vi "Temp from Voltage Calculator.vi"(8 "error in (no error)":errorcluster, 9 "Calibrations":dbl[](array[numeric]), 10 "Thermistor":T1, 11 "Data_Array":dbl[](array[numeric])) -> (1 "Temp Filtered":dbl[](array[numeric]), 2 "Temp":dbl[](array[numeric]), 3 "Time Read":timestamp[](array[timestamp]), 4 "error out":errorcluster[](array[cluster]))   [LabVIEW 2021]
uses:
  <vilib>/express/express arith-compare/Formula/XNode/ExpressFormulaBlockNode.xnode
  <vilib>/ptbypt/NI_PtbyPt.lvlib
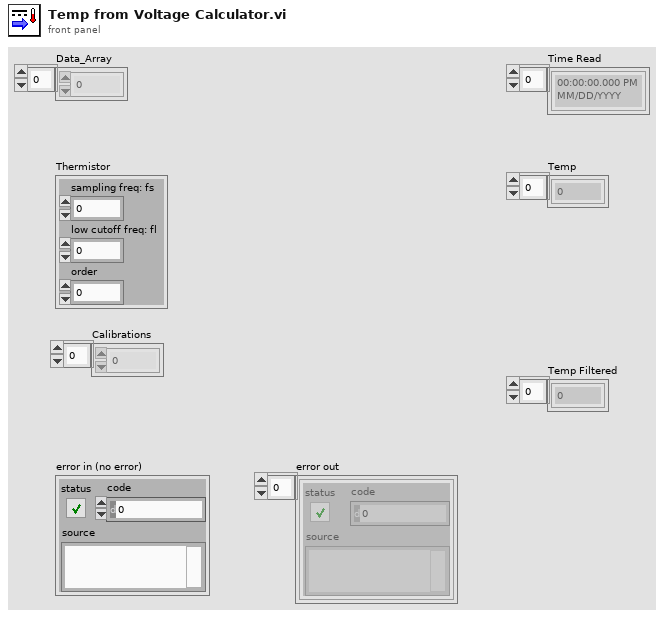
[diagram p1: front panel]
types:
  T1 = cluster{"sampling freq: fs":dbl, "low cutoff freq: fl":dbl, "order":i32}
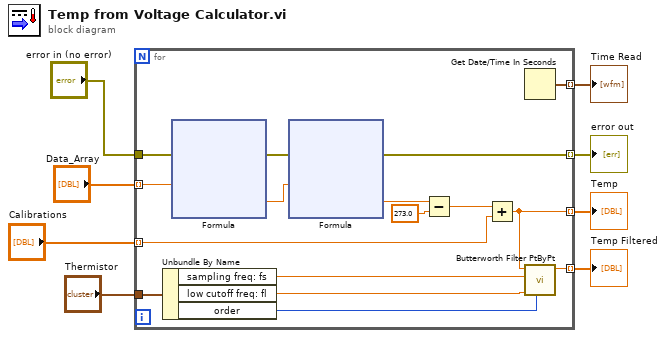
[diagram p0: block diagram]
diagram:
  n1 = for {
    tunnel: "Data_Array" -> [w19] mode=indexing
    tunnel: "Thermistor" -> [w18]
    tunnel: [w14] -> w4 mode=indexing
    tunnel: [w17] -> w8 mode=indexing
    tunnel: [w15] -> w7 mode=indexing
    tunnel: "error in (no error)" -> [w12]
    tunnel: [w10] -> w6 mode=indexing
    tunnel: "Calibrations" -> [w9] mode=indexing
    n2 = Unbundle By Name(w18) -> ("sampling freq: fs"=w23:dbl, "low cutoff freq: fl"=w22:dbl, "order"=w21:i32)
    n3 = xnode "Formula"("v"=w19, "error in (no error)"=w12) -> ("Result"=w13:dbl, "error out"=w11:errorcluster)
    n4 = xnode "Formula"("R"=w13, "error in (no error)"=w11) -> ("Result"=w20:dbl, "error out"=w10:errorcluster)
    n5 = Subtract(x=w20, y=273.0) -> (x-y=w16:dbl)
    n6 = Add(x=w16, y=w9) -> (x+y=w14:dbl)
    n7 = Get Date/Time In Seconds() -> (seconds since 1Jan1904=w15:timestamp)
    n8 = call <vilib>:"Butterworth Filter PtByPt.vi"("order"=w21, "low cutoff freq: fl"=w22, "sampling freq: fs"=w23, "x"=w14) -> ("Filtered x"=w17:dbl)  [unwired: 5 in, 1 out]
  }
  "Temp Filtered" <- w8
  "Time Read" <- w7
  "error out" <- w6
  "Temp" <- w4
